vi "Configure SPI Trigger Source.vi"(0 "VISA resource name":refnum<visa-resource-name>, 1 "SPI Data Width (8)":i32=8, 5 "Data Mask (0)":i32, 9 "Data Value (0)":i32, 11 "error in (no error)":errorcluster, 12 "Timeout (10E-6)":dbl=1e-05) -> (4 "VISA resource name out":refnum<visa-resource-name>, 15 "error out":errorcluster)   [LabVIEW 2017, in "Agilent 6000 Series.lvlib"]
doc: "This VI configures the SPI trigger. You specify the data width, value and mask with the SPI Data Width, Data Value and Data Mask parameters.\n\n<B>NOTE:</B>\n\nThis VI is only valid for 6000 Series models. An error will be thrown if this VI is run with 5000 Series scopes."
uses:
  <instrlib>/Agilent 6000 Series/Agilent 6000 Series.lvlib
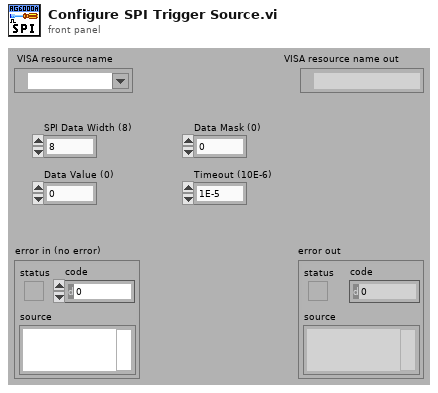
[diagram p1: front panel]
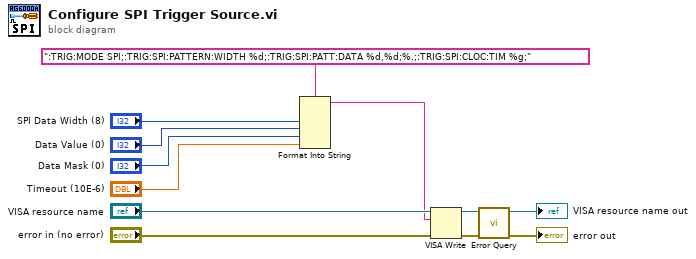
[diagram p0: block diagram]
diagram:
  n1 = Format Into String(format string=":TRIG:MODE SPI;:TRIG:SPI:PATTERN:WIDTH %d;:TRIG:SPI:PATT:DATA %d,%d;%.;:TRIG:SPI:CLOC:TIM %g;" ("Source Command"), "SPI Data Width (8)", "Data Value (0)", "Data Mask (0)", "Timeout (10E-6)") -> (resulting string=w5:string)  [unwired: 2 in, 1 out]
  n2 = VISA Write(VISA resource name="VISA resource name", write buffer=w5, error in (no error)="error in (no error)") -> (VISA resource name out=w8:refnum<visa-resource-name>, error out=w7:errorcluster)  [unwired: 1 out]
  n3 = call <instrlib>:"Error Query.vi"("error in (no error)"=w7, "VISA resource name"=w8) -> ("error out"=→"error out":errorcluster, "VISA resource name out"=→"VISA resource name out":refnum<visa-resource-name>)  [unwired: 6 in, 2 out]
